vi "Bind RPC GetMUXRelayInfo.vi"(11 "gRPCid server in":T3) -> (0 "error out":errorcluster, 1 "GetMUXRelayInfo Internal UE":T2, 2 "GetMUXRelayInfo gRPC UE":T1, 3 "gRPCid server out":T3)   [LabVIEW 2019, in "ctet_mux.lvlib" / "ctet_mux.lvclass"]
uses:
  ctet_mux.lvclass
  gRPC lvSupport/Server API/typeDefs/grpcId.ctl
  typeDefs/Server Internal Message UE.ctl
  typeDefs/Server Internal Message.ctl
  gRPC lvSupport/Server API/typeDefs/gRPCId Cluster UE.ctl
  gRPC lvSupport/Server API/typeDefs/gRPCId Cluster.ctl
  616620f9-6bbe-466a-af51-04bcc3596ea0.vi
  gRPC lvSupport/Server API/Server/Get Server DLL Path.vi
  gRPC lvSupport/gprc-lvsupport.lvlib
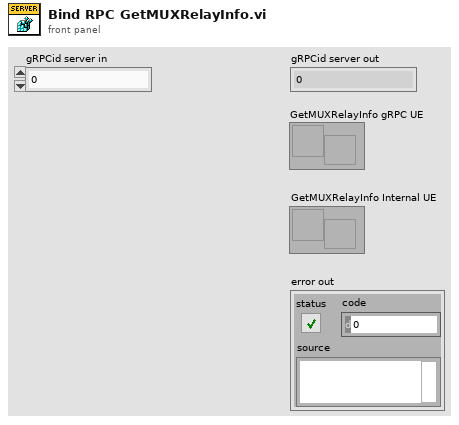
[diagram p1: front panel]
types:
  T1 = typedef "ctet_mux.lvlib/gprc-lvsupport.lvlib/gRPCId Cluster UE.ctl" = refnum<user-event>
  T2 = typedef "ctet_mux.lvlib/ctet_mux.lvclass/Server Internal Message UE.ctl" = refnum<user-event>
  T3 = typedef "ctet_mux.lvlib/gprc-lvsupport.lvlib/grpcId.ctl" = u64
  T4 = typedef "ctet_mux.lvlib/ctet_mux.lvclass/Server Internal Message.ctl" = cluster{"Command":string, "Data":variant}
  T5 = typedef "ctet_mux.lvlib/gprc-lvsupport.lvlib/gRPCId Cluster.ctl" = cluster{"gRPCid":T3}
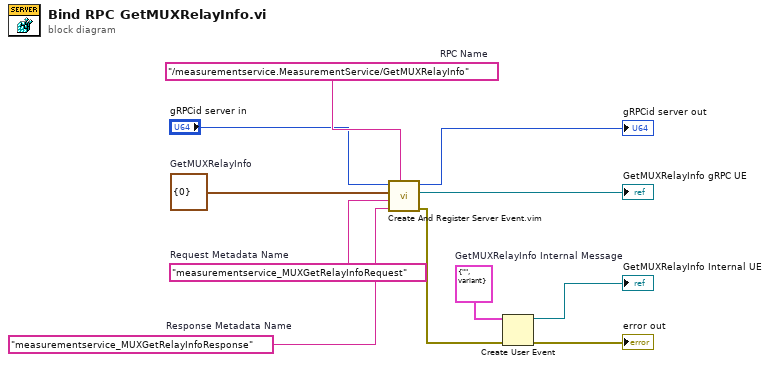
[diagram p0: block diagram]
diagram:
  w5 = T4 {"Command"="", "Data"=variant}  # GetMUXRelayInfo Internal Message
  w8 = "measurementservice_MUXGetRelayInfoResponse"  # Response Metadata Name
  w11 = T5 {"gRPCid"=0}  # GetMUXRelayInfo
  w9 = "measurementservice_MUXGetRelayInfoRequest"  # Request Metadata Name
  w10 = "/measurementservice.MeasurementService/GetMUXRelayInfo"  # RPC Name
  n1 = call "Create And Register Server Event.vim"("Method name"=w10, "Response Metadata Name"=w8, "Request Metadata Name"=w9, "event in"=w11, "gRPCid server in"="gRPCid server in") -> ("error out"=w4:errorcluster, "event"=→"GetMUXRelayInfo gRPC UE":refnum<user-event>, "gRPCid server out"=→"gRPCid server out":T3)  [unwired: 4 in]
  n2 = Create User Event(user event datatype=w5, error in=w4) -> (user event=→"GetMUXRelayInfo Internal UE":refnum<user-event>, error out=→"error out":errorcluster)
